vi "LaserCal-V to mW.vi"(0 "I-O":T1, 5 "Volts":dbl, 7 "Pulse width (us)":dbl, 9 "Pulse rate (Hz)":dbl, 11 "error in (no error)":errorcluster) -> (4 "Power (mW)":dbl, 15 "error out":errorcluster)   [LabVIEW 2020]
uses:
  42eadffc-ba4b-45d7-9f8f-eaa7c7697714.vi
  571ab1ba-4693-40e0-b1eb-368b057acf5f.vi
  c31a5c10-ecb5-4e74-8d8b-4da05ce192f9.vi
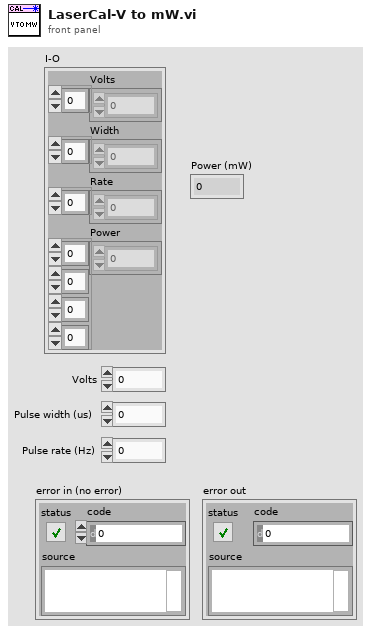
[diagram p1: front panel]
types:
  T1 = cluster{"Volts":dbl[], "Width":dbl[], "Rate":dbl[], "Power":dbl[][][][]}
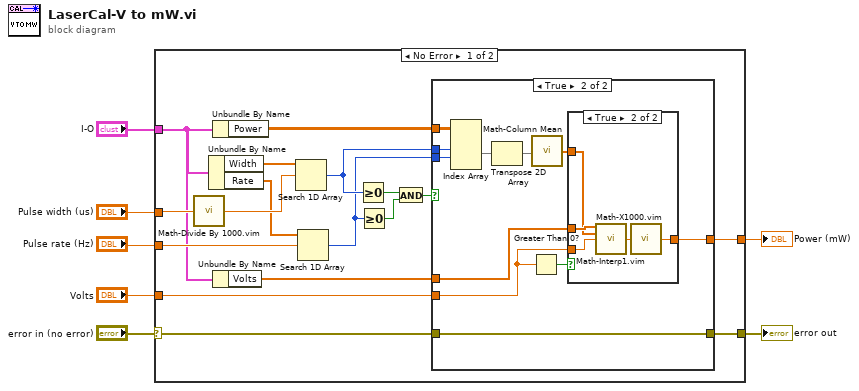
[diagram p0: block diagram]
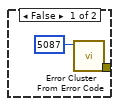
[diagram p2: hidden frame]
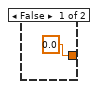
[diagram p3: hidden frame]
diagram:
  n1 = case shown="No Error" "error in (no error)" {
    selector: "error in (no error)" -> [w9 w44]
    tunnel: [w8 w44] -> w5
    tunnel: "Pulse width (us)" -> [w24 _]
    tunnel: "Pulse rate (Hz)" -> [w20 _]
    tunnel: [w15 _] -> w1
    tunnel: "I-O" -> [w18 _]
    tunnel: "Volts" -> [w16 _]
    frame No Error {
      n2 = call "Math-Divide By 1000.vim"("X"=w24) -> ("1000X"=w22:dbl)
      n3 = Unbundle By Name(w18) -> ("Width"=w23:dbl[], "Rate"=w21:dbl[])
      n4 = Unbundle By Name(w18) -> ("Power"=w19:dbl[][][][])
      n5 = Unbundle By Name(w18) -> ("Volts"=w17:dbl[])
      n6 = Search 1D Array(1D array=w23, element=w22) -> (index of element=w14:i32)  [unwired: 1 in]
      n7 = Search 1D Array(1D array=w21, element=w20) -> (index of element=w13:i32)  [unwired: 1 in]
      n8 = Greater Or Equal To 0?(x=w14) -> (x >= 0?=w12:bool)
      n9 = Greater Or Equal To 0?(x=w13) -> (x >= 0?=w11:bool)
      n10 = And(x=w12, y=w11) -> (x .and. y?=w10:bool)
      n11 = case shown="True" w10 {
        tunnel: w19 -> [_ w37]
        tunnel: w17 -> [_ w36]
        tunnel: [_ w31] -> w15
        tunnel: w16 -> [_ w32]
        tunnel: w14 -> [_ w35]
        tunnel: w13 -> [_ w34]
        tunnel: w9 -> [_ w30]
        tunnel: [w26 w30] -> w8
        frame False {
          n12 = call <vilib>:"Error Cluster From Error Code.vi"("error code (0)"=5087) -> ("error out"=w26:errorcluster)  [unwired: 8 in]
        }
        frame True {
          n13 = Index Array(array=w37, index (dim 1)=w35, index (dim 2)=w34) -> (element=w29:dbl[][])  [unwired: 2 in]
          n14 = Transpose 2D Array(2D array=w29) -> (transposed array=w27:dbl[][])
          n15 = Greater Than 0?(x=w32) -> (x > 0?=w33:bool)
          n16 = call "Math-Column Mean.vi"("2D Array"=w27) -> ("Column means"=w28:dbl[])
          n17 = case shown="True" w33 {
            tunnel: w36 -> [_ w41]
            tunnel: [0.0 ("V") w39] -> w31
            tunnel: w32 -> [_ w42]
            tunnel: w28 -> [_ w40]
            frame False {
            }
            frame True {
              n18 = call "Math-Interp1.vim"("X"=w41, "Y"=w40, "U"=w42) -> ("V"=w43:dbl)  [unwired: 12 in]
              n19 = call "Math-X1000.vim"("X"=w43) -> ("1000X"=w39:dbl)
            }
          }
        }
      }
    }
    frame Error {
    }
  }
  "Power (mW)" <- w1
  "error out" <- w5
